vi "trio_read_axis.vi"(6 "Error/Warning":bool, 7 "Axis":i16, 8 "error in (no error)":errorcluster, 9 "Variable":string, 10 "reference in":refnum<k7>) -> (0 "error out":errorcluster, 2 "Value":dbl, 3 "GetAxisVariable":bool)   [LabVIEW 2017]
uses:
  <instrlib>/Trio Motion/Trio Motion Library.lvlib
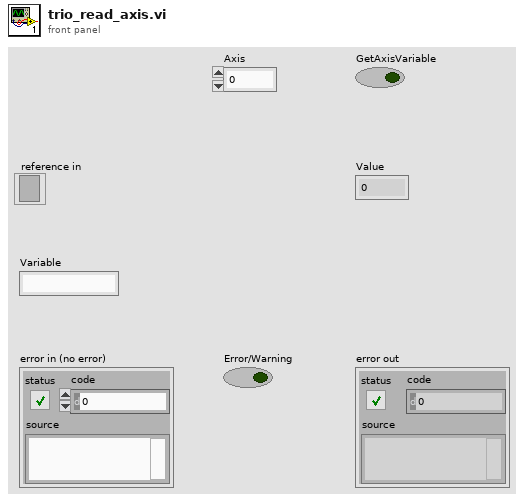
[diagram p1: front panel]
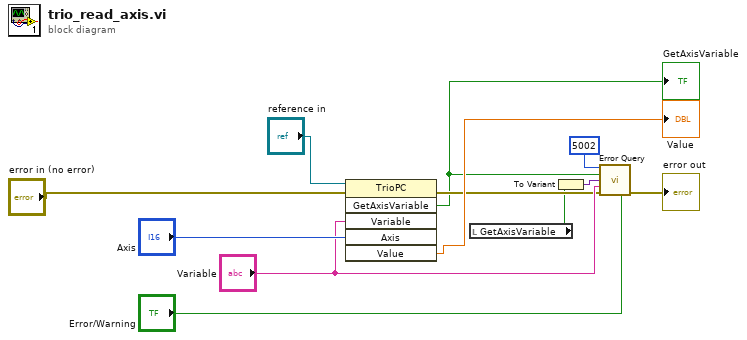
[diagram p0: block diagram]
diagram:
  n1 = invoke on="Invoke Node" class="TrioPC" method="GetAxisVariable"(reference="reference in", error in="error in (no error)", "Variable"="Variable", "Axis"="Axis") -> (error out=w4:errorcluster, "GetAxisVariable"=w2:bool, "Value"=→"Value":dbl)  [unwired: 2 in, 3 out]
  "GetAxisVariable" <- w2
  n2 = local read "GetAxisVariable"() -> (w1:bool)
  n3 = To Variant(anything=w1) -> (Variant=w6:variant)
  n4 = call <instrlib>:"Error Query.vi"("error code (0)"=5002, "State"=w2, "Command"=w6, "Parameter Name"="Variable", "error in (no error)"=w4, "Error/Warning (Error)"="Error/Warning") -> ("error out"=→"error out":errorcluster)  [unwired: 9 in]
